vi "ParseVersionString.vi"(5 "delimiter":string=".", 9 "version string":string) -> (3 "fixed version string":string, 4 "Version":T1)   [LabVIEW 2014, in "Raspberry Pi Compatible Compiler for LabVIEW.lvlib" / "RasPiDownloader.lvlib"]
uses:
  RasPiDownloader.lvlib
  RuntimeVersion.ctl
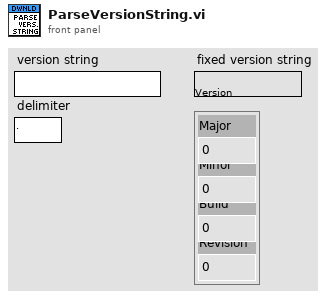
[diagram p1: front panel]
types:
  T1 = typedef "Raspberry Pi Compatible Compiler for LabVIEW.lvlib/RasPiDownloader.lvlib/RuntimeVersion.ctl" = cluster{"Major":i32, "Minor":i32, "Build":i32, "Revision":i32}
  T2 = cluster{"[0]":i32, "[1]":i32, "[2]":i32, "[3]":i32}
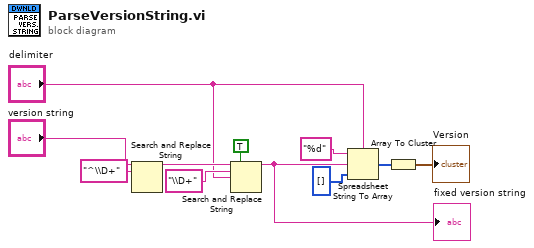
[diagram p0: block diagram]
diagram:
  n1 = Search and Replace String(input string="version string", search string="^\\D+") -> (result string=w9:string)  [unwired: 6 in, 3 out]
  n2 = Search and Replace String(replace all?=TRUE ("replace all? (F)"), input string=w9, search string="\\D+", replace string="delimiter") -> (result string=w4:string)  [unwired: 4 in, 3 out]
  "fixed version string" <- w4
  n3 = Spreadsheet String To Array(delimiter (Tab)="delimiter", format string="%d", spreadsheet string=w4, array type (2D Dbl)=i32[] []) -> (array=w3:i32[])
  n4 = Array To Cluster(array=w3) -> (cluster=→"Version":T2)
